vi "getObjectRefs.vi"(6 "type(ClassName)":string="Wire", 8 "error in (no error)":errorcluster, 11 "BlockDiagram in":refnum<class "AbstractDiagram.lvclass">) -> (0 "error out":errorcluster, 2 "refs":refnum<vi>[](array[refnum]), 3 "BlockDiagram out":refnum<class "AbstractDiagram.lvclass">)   [LabVIEW 2023, in "TLC_Scripto.lvlib" / "AbstractDiagram.lvclass"]
uses:
  AbstractDiagram.lvclass
  Read abstractDiagramRef.vi
  AbstractDiagram.lvclass/AbstractDiagram.ctl
  TLC_Scripto.lvlib
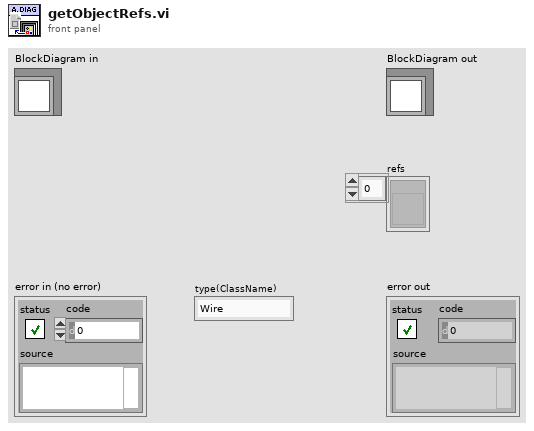
[diagram p1: front panel]
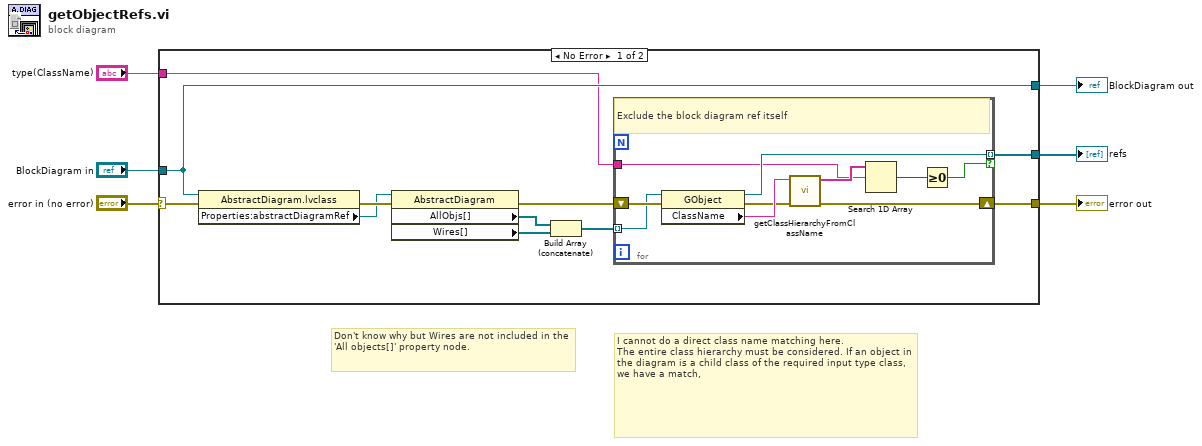
[diagram p0: block diagram]
diagram:
  # "Don't know why but Wires are not included in the 'All objects[]' property node."
  # "I cannot do a direct class name matching here.\nThe entire class hierarchy must be considered. If an object in the diagram is a child class of the required input type class, we have a match,"
  n1 = case shown="No Error" "error in (no error)" {
    selector: "error in (no error)" -> [w15 w29]
    tunnel: [w10 w29] -> w5
    tunnel: [w17 w28] -> w3
    tunnel: "BlockDiagram in" -> [w17 w28]
    tunnel: "type(ClassName)" -> [w12 _]
    tunnel: [w13 _] -> w1
    frame No Error {
      n2 = property class="AbstractDiagram.lvclass"(reference=w17, error in=w15) -> (error out=w16:errorcluster, "Properties:abstractDiagramRef"=w14:refnum<vi>)  [unwired: 1 out]
      n3 = property on="Property Node" class="AbstractDiagram"(reference=w14, error in=w16) -> (error out=w11:errorcluster, "AllObjs[]"=w7:refnum<vi>[], "Wires[]"=w9:refnum<vi>[])  [unwired: 1 out]
      n4 = Build Array (concatenate)(w7, w9) -> (w8:refnum<vi>[])
      n5 = for {
        tunnel: [w26] -> w13 mode=indexing if=w20
        tunnel: w8 -> [w25] mode=indexing
        tunnel: w12 -> [w22]
        shift-right: [w18] -> w10
        shift-left: w11 -> [w27]
        # "Exclude the block diagram ref itself"
        n6 = property on="Property Node" class="GObject"(reference=w25, error in=w27) -> (reference out=w26:refnum<vi>, error out=w19:errorcluster, "ClassName"=w24:string)
        n7 = call "getClassHierarchyFromClassName.vi"("error in (no error)"=w19, "className"=w24) -> ("error out"=w18:errorcluster, "hierarchy"=w23:string[])  [unwired: 8 in]
        n8 = Search 1D Array(1D array=w23, element=w22) -> (index of element=w21:i32)  [unwired: 1 in]
        n9 = Greater Or Equal To 0?(x=w21) -> (x >= 0?=w20:bool)
      }
    }
    frame Error {
    }
  }
  "error out" <- w5
  "BlockDiagram out" <- w3
  "refs" <- w1
